vi "Checkout.vi"(8 "error in (no error)":errorcluster, 9 "Timeout (-1)":dbl[unit], 11 "Object Reference":refnum<class "CS++Reference.lvclass">) -> (0 "error out":errorcluster, 1 "timed out?":bool, 2 "Object":refnum<class "CS++Base.lvclass">, 3 "Object Reference out":refnum<class "CS++Reference.lvclass">)   [LabVIEW 2012, in "CS++BaseClasses.lvlib" / "CS++Reference.lvclass"]
doc: "Checkout object from Reference."
uses:
  CS++Reference.lvclass
  Base/CS++Base.lvclass
  CS++Reference.lvclass/CS++Reference.ctl
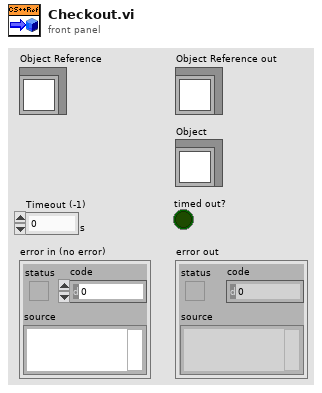
[diagram p1: front panel]
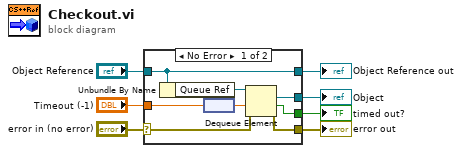
[diagram p0: block diagram]
diagram:
  n1 = case shown="No Error" "error in (no error)" {
    selector: "error in (no error)" -> [w13 w17]
    tunnel: [w10 w17] -> w6
    tunnel: [w15 w16] -> w4
    tunnel: "Object Reference" -> [w15 w16]
    tunnel: "Timeout (-1)" -> [w11 _]
    tunnel: [w9 _] -> w2
    tunnel: [w8 _] -> w1
    frame No Error {
      n2 = Unbundle By Name(w15) -> ("Queue Ref"=w14:refnum<queue>)
      n3 = node(w11) -> (w12:dbl)
      n4 = Dequeue Element(queue=w14, timeout in ms (-1)=w12, error in (no error)=w13) -> (element=w9:refnum<class "CS++Base.lvclass">, timed out?=w8:bool, error out=w10:errorcluster)  [unwired: 1 out]
    }
    frame Error {
    }
  }
  "error out" <- w6
  "Object Reference out" <- w4
  "Object" <- w2
  "timed out?" <- w1
